vi "PolyFitNaN.vi"(11 "Data":dbl[](array[numeric])) -> (2 "Polynomial Coefficients":dbl[](array[numeric]), 3 "Best Polynomial Fit":dbl[](array[numeric]))   [LabVIEW 2014, in "Head Impulse Fit.lvclass"]
uses:
  Head Impulse Fit.lvclass
  <vilib>/Analysis/6fits.llb/General Linear Fit Algorithm.ctl
  <vilib>/Analysis/1siggen.llb/Ramp Pattern by Samples.vi
  <vilib>/Analysis/polynomials.llb/1D Polynomial Evaluation (DBL).vi
  <vilib>/Analysis/NI_AALPro.lvlib
  <vilib>/Analysis/NI_AALBase.lvlib
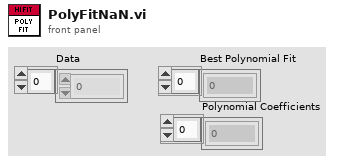
[diagram p1: front panel]
types:
  T1 = typedef "NI_AALPro.lvlib/General Linear Fit Algorithm.ctl" = u16
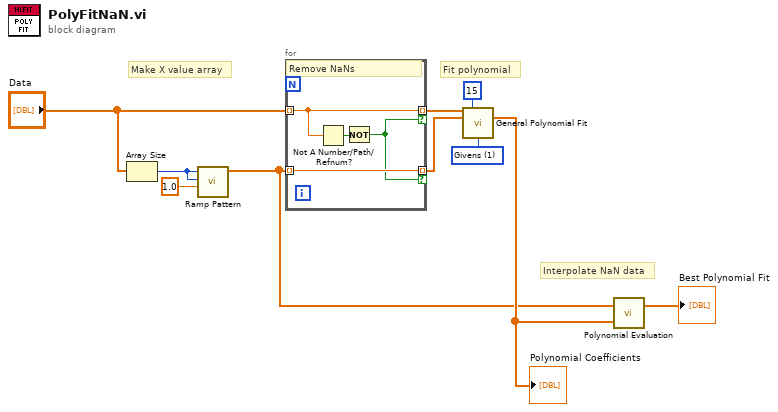
[diagram p0: block diagram]
diagram:
  w5 = T1 1 items=["SVD", "Givens", "Givens2", "Householder", "LU Decomposition", "Cholesky", "SVD for Rank Deficient H"] ("algorithm")
  # "Interpolate NaN data"
  # "Make X value array"
  # "Fit polynomial"
  n1 = Array Size(array="Data") -> (size(s)=w8:i32)
  n2 = call-poly <vilib>:"Ramp Pattern.vi"("start"=1.0, "end"=w8, "samples"=w8) -> ("Ramp Pattern"=w2:dbl[])  [unwired: 7 in, 1 out]
  n3 = for {
    tunnel: "Data" -> [w14] mode=indexing
    tunnel: w2 -> [w13] mode=indexing
    tunnel: [w14] -> w10 mode=indexing if=w11
    tunnel: [w13] -> w9 mode=indexing if=w11
    # "Remove NaNs"
    n4 = Not A Number/Path/Refnum?(number/path/refnum=w14) -> (NaN/Path/Refnum?=w12:bool)
    n5 = Not(x=w12) -> (.not. x?=w11:bool)
  }
  n6 = call <vilib>:"General Polynomial Fit.vi"("Y"=w10, "polynomial order"=15, "X"=w9, "algorithm"=w5) -> ("Polynomial Coefficients"=w3:dbl[])  [unwired: 8 in, 3 out]
  "Polynomial Coefficients" <- w3
  n7 = call-poly <vilib>:"Polynomial Evaluation.vi"("P(x)"=w3, "A"=w2) -> ("P(A)"=→"Best Polynomial Fit":dbl[])  [unwired: 1 out]
